vi "Stop Core.vi"(10 "final error code":i32, 11 "Classic Monitor in":refnum<class "Classic Monitor.lvclass">) -> (3 "Classic Monitor out":refnum<class "Classic Monitor.lvclass">)   [LabVIEW 2020, in "Monitored Actor.lvlib" / "Classic Monitor.lvclass"]
doc: "(<B>Filename</B>: Actor Framework.lvlib:Actor.lvclass:Stop Core.vi)\n\nDefines what the actor does before it stops. Use the <B>final error code</B> input to determine whether the actor shut down in response to an error.\n\nBy default, this method does nothing. A descendant class may override it to define behavior, such as shutting down any processes the actor initiated in its override of the Actor Core method."
uses:
  <vilib>/MGI/Monitored Actor/Classic Monitor/Monitor/Monitor Actor/Classic Monitor.lvclass
  <vilib>/MGI/Monitored Actor/Classic Monitor/Monitor/Monitor Actor/Classic Monitor.lvclass/Classic Monitor.ctl
  <vilib>/ActorFramework/Message Enqueuer/Message Enqueuer.lvclass/Message Enqueuer.ctl
  <vilib>/ActorFramework/Message Enqueuer/Enqueue.vi
  <vilib>/ActorFramework/Stop Msg/Stop Msg.lvclass
  C:/Program Files/National Instruments/LabVIEW 2020/vi.lib/ActorFramework/Message/Message.lvclass
  <vilib>/ActorFramework/Message Priority Queue/Priority Enqueue.vi
  <vilib>/MGI/Monitored Actor/Actor Monitor/Actor Monitor/Actor Monitor.lvclass
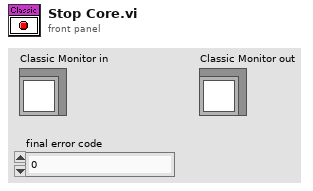
[diagram p1: front panel]
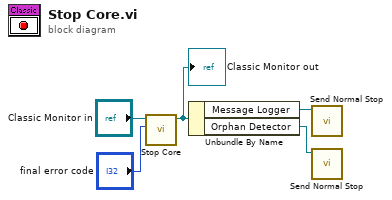
[diagram p0: block diagram]
diagram:
  n1 = call-parent "Stop Core.vi"("final error code"="final error code", "Actor in"="Classic Monitor in") -> ("Actor out"=w3:refnum<class "Classic Monitor.lvclass">)  [unwired: 9 in]
  "Classic Monitor out" <- w3
  n2 = Unbundle By Name(w3) -> ("Message Logger"=w2:refnum<class "Message Enqueuer.lvclass">, "Orphan Detector"=w1:refnum<class "Message Enqueuer.lvclass">)
  n3 = call <vilib>:"Send Normal Stop.vi"("Message Enqueuer"=w2) -> ()  [unwired: 10 in, 1 out]
  n4 = call <vilib>:"Send Normal Stop.vi"("Message Enqueuer"=w1) -> ()  [unwired: 10 in, 1 out]
